vi "event and random number.vi"() -> ()   [LabVIEW 2023]
uses:
  <vilib>/numeric/Random Number (Range) U64.vi
  <vilib>/numeric/sub_Random U32.vi
panel:
  in  "stop":bool
  in  "OK Button":bool
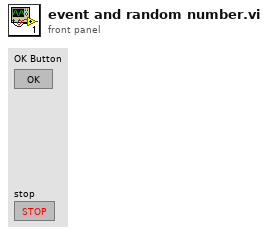
[diagram p1: front panel]
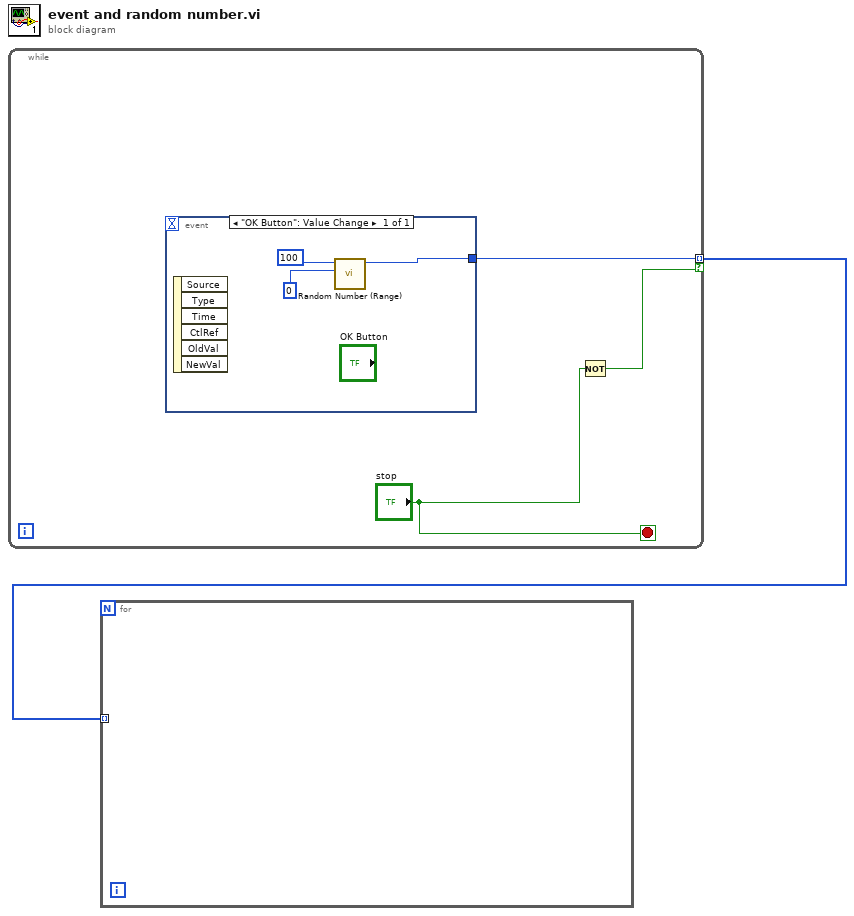
[diagram p0: block diagram]
diagram:
  n1 = while {
    tunnel: [w4] -> w1 mode=indexing if=w2
    stop <- "stop" stop-if-true
    n2 = event shown="[0] \"OK Button\": Value Change" {
      selector: _ -> [_]
      dyn-events: _ -> [_]
      timeout: _ -> [_]
      tunnel: [w5] -> w4
      event "OK Button": Value Change {
        n3 = event-data() -> ()  [unwired: 1 in, 6 out]
        n4 = call-poly <vilib>:"Random Number (Range).vi"("lower bound (0)"=u64 0, "upper bound (100)"=u64 100) -> ("number"=w5:u64)  [unwired: 9 in]
      }
    }
    n5 = Not(x="stop") -> (.not. x?=w2:bool)
  }
  n6 = for {
    tunnel: w1 -> [_] mode=indexing
  }
